vi "Close.vi"(8 "error in":errorcluster, 11 "Iso Measurement in":refnum<class "Iso Measurement.lvclass">) -> (0 "error out":errorcluster, 3 "Iso Measurement out":refnum<class "Iso Measurement.lvclass">)   [LabVIEW 2023, in "Iso Measurement.lvclass"]
uses:
  Iso Measurement.lvclass
  Iso Measurement.lvclass/Iso Measurement.ctl
  <vilib>/ADAS Replay HIL/AdasHilServices/AdasHilChannelServices.lvlib
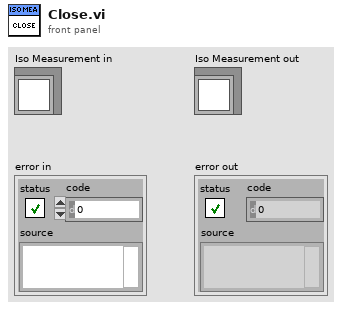
[diagram p1: front panel]
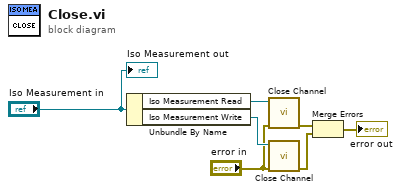
[diagram p0: block diagram]
diagram:
  n1 = Unbundle By Name("Iso Measurement in") -> ("Iso Measurement Read"=w6:refnum<k21>, "Iso Measurement Write"=w5:refnum<k21>)
  n2 = call <vilib>:"Close Channel.vi"("error in"="error in", "ADAS HIL Channel"=w6) -> ("error out"=w7:errorcluster)  [unwired: 9 in]
  n3 = call <vilib>:"Close Channel.vi"("error in"="error in", "ADAS HIL Channel"=w5) -> ("error out"=w2:errorcluster)  [unwired: 9 in]
  n4 = Merge Errors(w7, w2) -> (→"error out":errorcluster)
  "Iso Measurement out" <- "Iso Measurement in"
